vi "AIs.vi"() -> ()   [LabVIEW 2023]
uses:
  <instrlib>/HandsOnPi2040/cti-drivers-lv-visa-main/CTI-Visa/Identity.ctl
  <instrlib>/HandsOnPi2040/Public/AnaIns.ctl
  <instrlib>/HandsOnPi2040/HandsOnPi2040.lvlib
  <instrlib>/HandsOnPi2040/cti-drivers-lv-visa-main/CTI-Visa/CTI-Visa.lvlib
panel:
  out "Identity":T1
  out "27":i16
  out "26":i16
  out "error out":errorcluster
  in  "stop":bool
  out "Value":u16(graph)
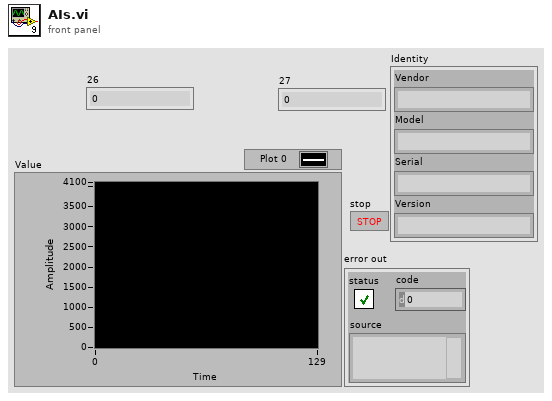
[diagram p1: front panel]
types:
  T1 = typedef "CTI-Visa.lvlib/Identity.ctl" = cluster{"Vendor":string, "Model":string, "Serial":string, "Version":string}
  T2 = typedef "HandsOnPi2040.lvlib/AnaIns.ctl" = enum16{"No AI - Error", "AI1 (GPIO26)", "AI2 (GPIO27)"}
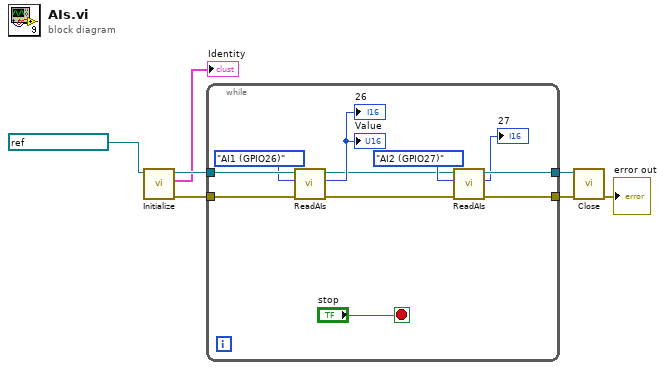
[diagram p0: block diagram]
diagram:
  n1 = call <instrlib>:"Initialize.vi"("VISA resource name"=refnum<visa-resource-name> "ASRL5::INSTR") -> ("error out"=w6:errorcluster, "Identity"=→"Identity":T1, "VISA resource name out"=w5:refnum<visa-resource-name>)  [unwired: 8 in]
  n2 = while {
    tunnel: [w9] -> w7
    tunnel: w6 -> [w18]
    tunnel: w5 -> [w17]
    tunnel: [w10] -> w4
    stop <- "stop" stop-if-true
    n3 = call <instrlib>:"ReadAIs.vi"("error in (no error)"=w18, "Analog Inputs"=AnaIns."AI1 (GPIO26)", "VISA resource name"=w17) -> ("error out"=w11:errorcluster, "Value"=→"Value" →"26":u16, "VISA resource name out"=w12:refnum<visa-resource-name>)  [unwired: 6 in]
    n4 = call <instrlib>:"ReadAIs.vi"("error in (no error)"=w11, "Analog Inputs"=AnaIns."AI2 (GPIO27)", "VISA resource name"=w12) -> ("error out"=w9:errorcluster, "Value"=→"27":u16, "VISA resource name out"=w10:refnum<visa-resource-name>)  [unwired: 6 in]
  }
  n5 = call <instrlib>:"Close.vi"("error in (no error)"=w7, "VISA resource name"=w4) -> ("error out"=→"error out":errorcluster)  [unwired: 9 in]
